vi "new_CTR_DAQModuleConfigs.vi"(8 "error in":errorcluster, 10 "Modules":T1(array[cluster]), 11 "node in":refnum<k20>) -> (0 "error out":errorcluster={"status"=TRUE, "code"=-2633, "source"="Property Node (arg 1) in NI_XML.lvlib:Get Node Text Content.vi->CTR_ControlNodeConfigs.vi->CTR_ReadXML_Config.vi->CTRnode.vi"}, 2 "Modules":T1(array[cluster]), 3 "node out":refnum<k20>)   [LabVIEW 2024]
uses:
  <vilib>/xml/Close Reference(Node).vi
  <vilib>/xml/NI_XML.lvlib
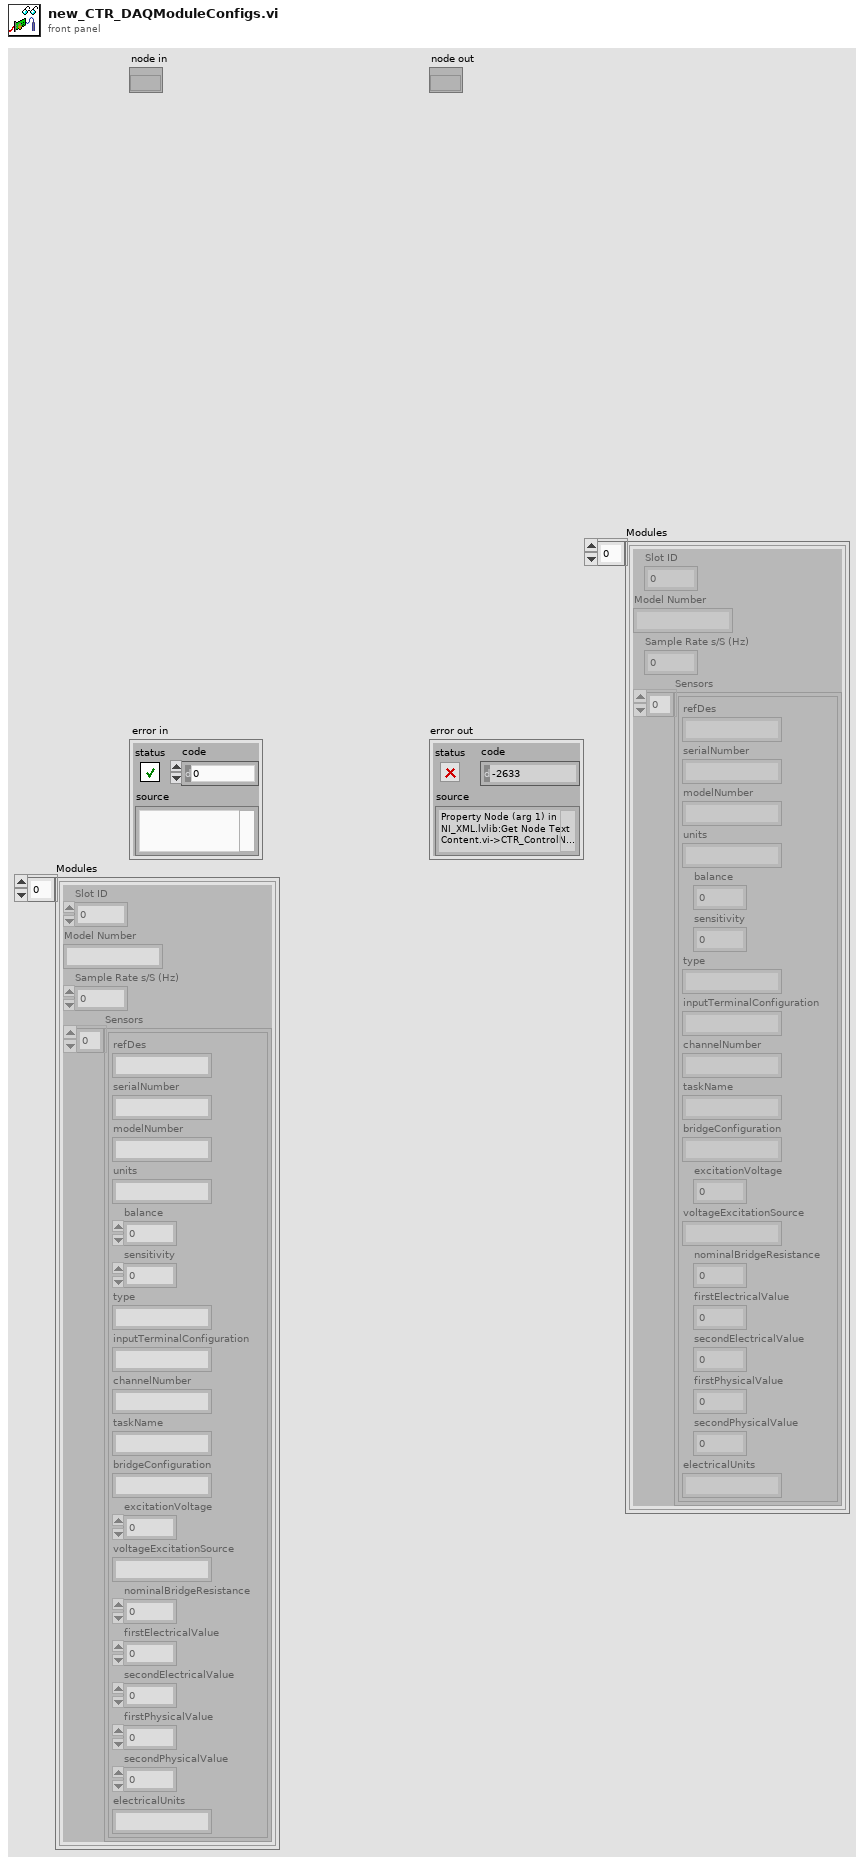
[diagram p1: front panel]
types:
  T1 = cluster{"Slot ID":i32, "Model Number":string, "Sample Rate s/S (Hz)":dbl, "Sensors":cluster{"refDes":string, "serialNumber":string, "modelNumber":string, "units":string, "balance":dbl, "sensitivity":dbl, "type":string, "inputTerminalConfiguration":string, "channelNumber":string, "taskName":string, "bridgeConfiguration":string, "excitationVoltage":dbl, "voltageExcitationSource":string, "nominalBridgeResistance":dbl, "firstElectricalValue":dbl, "secondElectricalValue":dbl, "firstPhysicalValue":dbl, "secondPhysicalValue":dbl, "electricalUnits":string}[]}[]
  T2 = cluster{"Slot ID":i32, "Model Number":string, "Sample Rate s/S (Hz)":dbl, "Sensors":cluster{"refDes":string, "serialNumber":string, "modelNumber":string, "units":string, "balance":dbl, "sensitivity":dbl, "type":string, "inputTerminalConfiguration":string, "channelNumber":string, "taskName":string, "bridgeConfiguration":string, "excitationVoltage":dbl, "voltageExcitationSource":string, "nominalBridgeResistance":dbl, "firstElectricalValue":dbl, "secondElectricalValue":dbl, "firstPhysicalValue":dbl, "secondPhysicalValue":dbl, "electricalUnits":string}[]}
  T3 = cluster{"[0]":string, "[1]":string, "[2]":string}
  T4 = cluster{"refDes":string, "serialNumber":string, "modelNumber":string, "units":string, "balance":dbl, "sensitivity":dbl, "type":string, "inputTerminalConfiguration":string, "channelNumber":string, "taskName":string, "bridgeConfiguration":string, "excitationVoltage":dbl, "voltageExcitationSource":string, "nominalBridgeResistance":dbl, "firstElectricalValue":dbl, "secondElectricalValue":dbl, "firstPhysicalValue":dbl, "secondPhysicalValue":dbl, "electricalUnits":string}[]
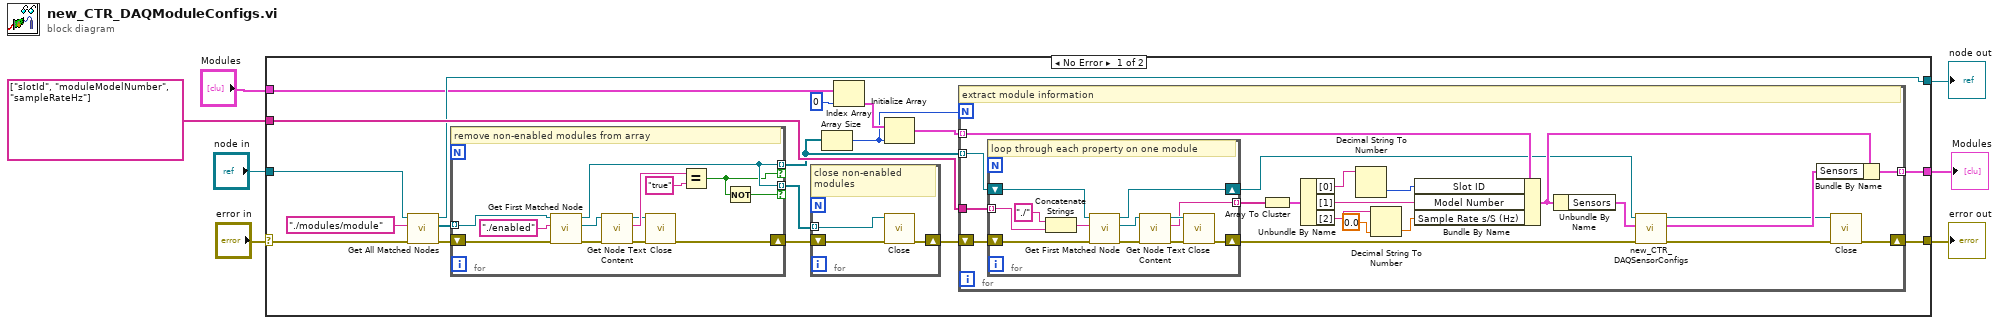
[diagram p0: block diagram]
diagram:
  n1 = case shown="No Error" "error in" {
    selector: "error in" -> [w25 w77]
    tunnel: [w24 w77] -> w6
    tunnel: "node in" -> [w22 w76]
    tunnel: string[] ["slotId", "moduleModelNumber", "sampleRateHz"] -> [w21 _]
    tunnel: [w13 w76] -> w7
    tunnel: "Modules" -> [w9 w75]
    tunnel: [w8 w75] -> w1
    frame No Error {
      n2 = call <vilib>:"Get All Matched Nodes.vi"("error in (no error)"=w25, "XPath expression"="./modules/module" ("string"), "node in"=w22) -> ("error out"=w17:errorcluster, "node result array"=w14:refnum<k20>[], "node out"=w13:refnum<k20>)  [unwired: 6 in]
      n3 = for {
        shift-right: [w33] -> w19
        shift-left: w17 -> [w34]
        tunnel: [w32] -> w15 mode=indexing if=w30
        tunnel: [w32] -> w18 mode=indexing if=w31
        tunnel: w14 -> [w29] mode=indexing
        # "remove non-enabled modules from array"
        n4 = call <vilib>:"Get First Matched Node.vi"("error in (no error)"=w34, "XPath expression"="./enabled", "node in"=w29) -> ("error out"=w37:errorcluster, "node result"=w38:refnum<k20>, "node out"=w32:refnum<k20>)  [unwired: 6 in]
        n5 = call <vilib>:"Get Node Text Content.vi"("error in (no error)"=w37, "node in"=w38) -> ("error out"=w39:errorcluster, "node text"=w41:string, "node out"=w40:refnum<k20>)  [unwired: 7 in]
        n6 = call-poly <vilib>:"Close.vi"("error in (no error)"=w39, "node"=w40) -> ("error out"=w33:errorcluster)  [unwired: 7 in]
        n7 = Equal?(x=w41, y="true" ("x")) -> (x = y?=w30:bool)
        n8 = Not(x=w30) -> (.not. x?=w31:bool)
      }
      n9 = for {
        tunnel: w18 -> [w28] mode=indexing
        shift-right: [w26] -> w16
        shift-left: w19 -> [w27]
        # "close non-enabled modules"
        n10 = call-poly <vilib>:"Close.vi"("error in (no error)"=w27, "node"=w28) -> ("error out"=w26:errorcluster)  [unwired: 7 in]
      }
      n11 = Array Size(array=w15) -> (size(s)=w11:i32)
      n12 = Index Array(array=w9, index=0) -> (element=w12:T2)
      n13 = Initialize Array(w12, w11) -> (w10:T1)
      n14 = for {
        N: w11 -> [_]
        shift-right: [w48] -> w24
        shift-left: w16 -> [w61]
        tunnel: w21 -> [w62]
        tunnel: w15 -> [w60] mode=indexing
        tunnel: w10 -> [w59] mode=indexing
        tunnel: [w50] -> w8 mode=indexing
        # "extract module information"
        n15 = for {
          tunnel: w62 -> [w68] mode=indexing
          shift-right: [w63] -> w46
          shift-left: w61 -> [w70]
          shift-right: [w65] -> w47
          shift-left: w60 -> [w66]
          tunnel: [w64] -> w58 mode=indexing
          # "loop through each property on one module"
          n16 = Concatenate Strings("./" ("string"), w68) -> (w67:string)
          n17 = call <vilib>:"Get First Matched Node.vi"("error in (no error)"=w70, "XPath expression"=w67, "node in"=w66) -> ("error out"=w74:errorcluster, "node result"=w73:refnum<k20>, "node out"=w65:refnum<k20>)  [unwired: 6 in]
          n18 = call <vilib>:"Get Node Text Content.vi"("error in (no error)"=w74, "node in"=w73) -> ("error out"=w72:errorcluster, "node text"=w64:string, "node out"=w71:refnum<k20>)  [unwired: 7 in]
          n19 = call-poly <vilib>:"Close.vi"("error in (no error)"=w72, "node"=w71) -> ("error out"=w63:errorcluster)  [unwired: 7 out]
        }
        n20 = Array To Cluster(array=w58) -> (cluster=w57:T3)
        n21 = Unbundle By Name(w57) -> ("[0]"=w55:string, "[1]"=w56:string, "[2]"=w53:string)
        n22 = Decimal String To Number(string=w55) -> (number=w54:i32)  [unwired: 2 in, 1 out]
        n23 = Decimal String To Number(string=w53, default (0L)=0.0) -> (number=w51:dbl)  [unwired: 1 in, 1 out]
        n24 = Bundle By Name(cluster=w59, "Slot ID"=w54, "Model Number"=w56, "Sample Rate s/S (Hz)"=w51) -> (w49:T2)
        n25 = Unbundle By Name(w49) -> ("Sensors"=w42:T4)
        n26 = call "new_CTR_DAQSensorConfigs.vi"("error in"=w46, "Sensors"=w42, "node in"=w47) -> ("error out"=w45:errorcluster, "Sensors"=w44:T4, "node out"=w43:refnum<k20>)  [unwired: 6 in]
        n27 = Bundle By Name(cluster=w49, "Sensors"=w44) -> (w50:T2)
        n28 = call-poly <vilib>:"Close.vi"("error in (no error)"=w45, "node"=w43) -> ("error out"=w48:errorcluster)  [unwired: 7 out]
      }
    }
    frame Error {
    }
  }
  "error out" <- w6
  "node out" <- w7
  "Modules" <- w1
